vi "Set_Dll_Data.vi"(8 "error in (no error)":errorcluster, 10 "data":T1, 11 "Class in":refnum<class "AB_DLL.lvclass">) -> (0 "error out":errorcluster, 3 "Class out":refnum<class "AB_DLL.lvclass">)   [LabVIEW 2020, in "AB_DLL.lvclass"]
uses:
  <vilib>/AppBuilder/AB_Classes/DLL/AB_DLL.lvclass
  <vilib>/AppBuilder/AB_Classes/DLL/AB_DLL.ctl
  <vilib>/AppBuilder/AB_Classes/DLL/AB_DLL.lvclass/AB_DLL.ctl
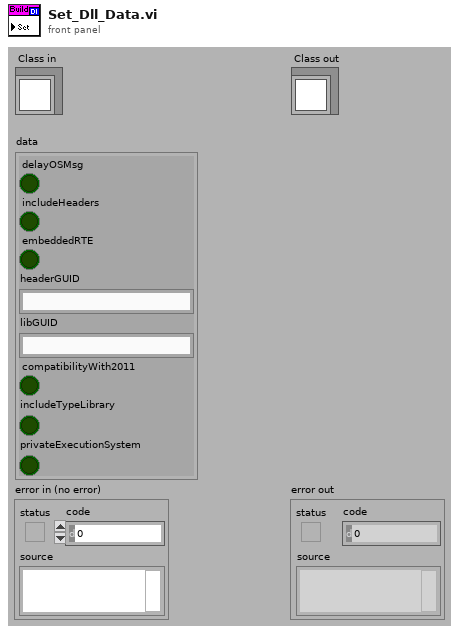
[diagram p1: front panel]
types:
  T1 = typedef "AB_DLL.ctl" = cluster{"delayOSMsg":bool, "includeHeaders":bool, "embeddedRTE":bool, "headerGUID":string, "libGUID":string, "compatibilityWith2011":bool, "includeTypeLibrary":bool, "privateExecutionSystem":bool}
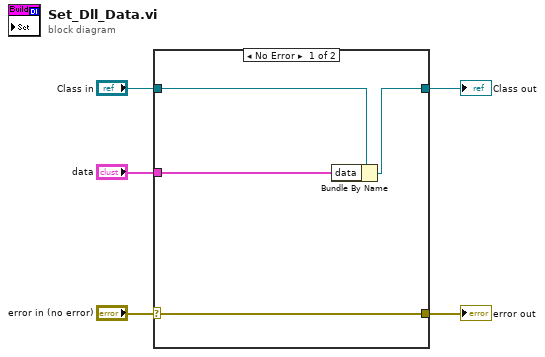
[diagram p0: block diagram]
diagram:
  n1 = case shown="No Error" "error in (no error)" {
    selector: "error in (no error)" -> [w9 w11]
    tunnel: [w9 w11] -> w4
    tunnel: [w6 w10] -> w2
    tunnel: "Class in" -> [w8 w10]
    tunnel: "data" -> [w7 _]
    frame No Error {
      n2 = Bundle By Name(cluster=w8, "data"=w7) -> (w6:refnum<class "AB_DLL.lvclass">)
    }
    frame Error {
    }
  }
  "Class out" <- w2
  "error out" <- w4
